vi "Client Test.vi"() -> ()   [LabVIEW 2018, in "OPC UA Total Client.lvlib"]
uses:
  OPC UA Total Client.lvlib
  OPC Tag Data.ctl
  <vilib>/OPCUA/controls/NodeIds.ctl
  <vilib>/OPCUA/controls/NodeId.ctl
  <vilib>/OPCUA/controls/Write Variant Request.ctl
  <vilib>/OPCUA/controls/Write Status.ctl
  support/Message Queue/Enqueue Message (Single).vi
  <vilib>/OPCUA/client/Multiple Write Variant.vi
  <vilib>/OPCUA/NI OPC UA Client.lvlib
  support/Message Queue/Message Queue.lvlib
  OPC UA.lvlib
panel:
  out "Tag Data":T1[](array[typedef])
  out "error out":errorcluster
  out "Object Cluster":T2
  in  "Numeric":dbl
  in  "Send":bool
  in  "Variable Ring":u16(ring) items=["Default", "ns=2;s=FD1.FD1:Density", "ns=2;s=FD1.FD1:FL_Temp", "ns=2;s=FD1.FD1:PID2Out", "ns=2;s=FD1.FD1:Pump_Flow", "ns=2;s=FD1.FD1:Input_Device_Disconnected", "ns=2;s=FD1.FD1:Output_Device_Disconnected"]
  in  "Object Ring":u16(ring) items=["Default", "Server", "FD1", "FD2", "FD3"]
  in  "security policy":T3
  in  "stop":bool
  out "Waveform Chart":i32(graph)
  in  "server endpoint URL":string="opc.tcp://10.131.1.22:4840"
  # "opc.tcp://10.131.1.22:4840"
  # "opc.tcp://127.0.0.1:49320"
  # "opc.tcp://AMRGROBJ07MYKD.amer.pfizer.com:49320"
  # "opc.tcp://AMRGROBJ07MYKD:49580"
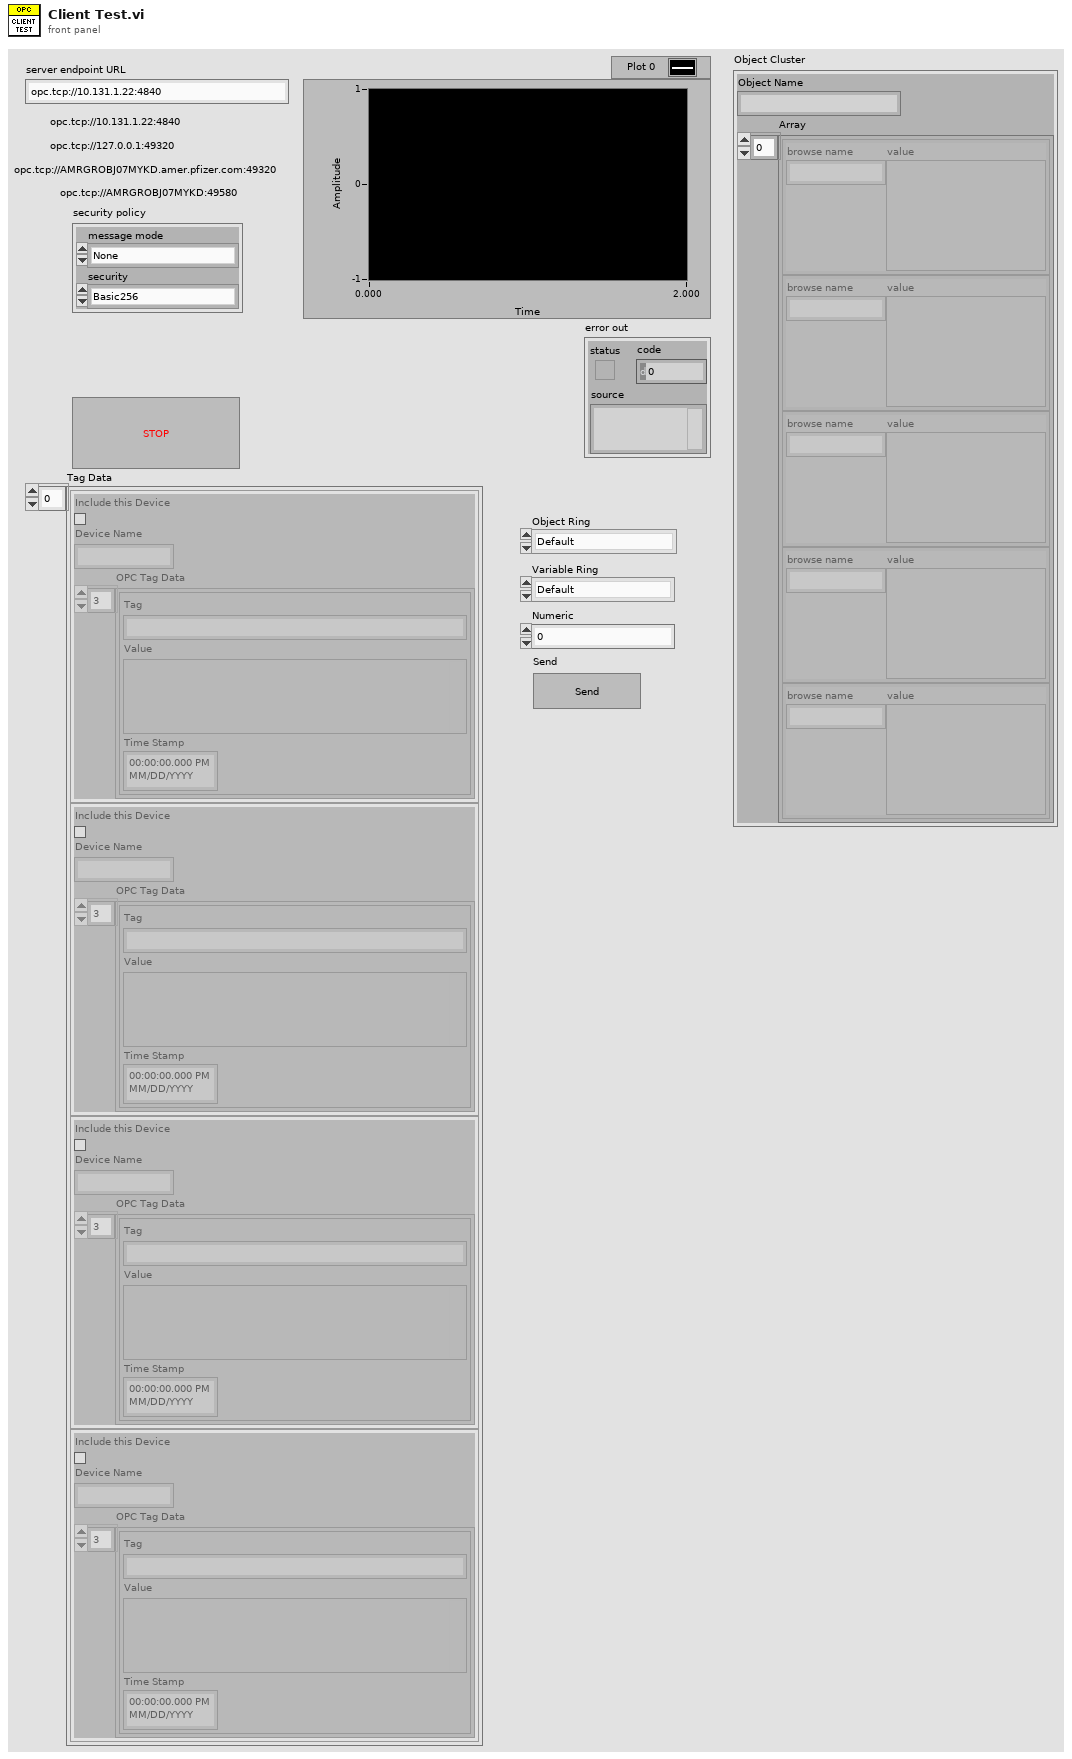
[diagram p1: front panel]
types:
  T1 = typedef "OPC UA.lvlib/OPC Tag Data.ctl" = cluster{"Include this Device":bool, "Device Name":string, "OPC Tag Data":cluster{"Tag":string, "Value":variant, "Time Stamp":timestamp}[]}
  T2 = cluster{"Object Name":string, "Array":cluster{"browse name":string, "value ":variant}[]}
  T3 = cluster{"message mode":enum16{"None", "Sign", "Sign and Encrypt"}, "security":enum16{"Basic256", "Basic128Rsa15"}}
  T4 = typedef "NodeIds.ctl" = T5[]
  T5 = typedef "NodeId.ctl" = string
  T6 = typedef "OPC UA Client Refnum.ctl" = refnum<k21>
  T7 = typedef "Subscription ID.ctl" = u32
  T8 = typedef "Write Variant Request.ctl" = cluster{"node ID":T5, "value":variant, "timestamp (current time)":timestamp, "node status":T9}
  T9 = typedef "Write Status.ctl" = u32
  T10 = typedef "Subscription Data Change.ctl" = cluster{"node ID":T5, " value":variant, "timestamp":timestamp, "data type":T11, "status code":T12}
  T11 = typedef "Data Type.ctl" = u16
  T12 = typedef "OPC UA StatusCode.ctl" = u32
  T13 = cluster{"Tag":string, "Value":variant, "Time Stamp":timestamp}[]
  T14 = cluster{"Tag":string, "Value":variant, "Time Stamp":timestamp}
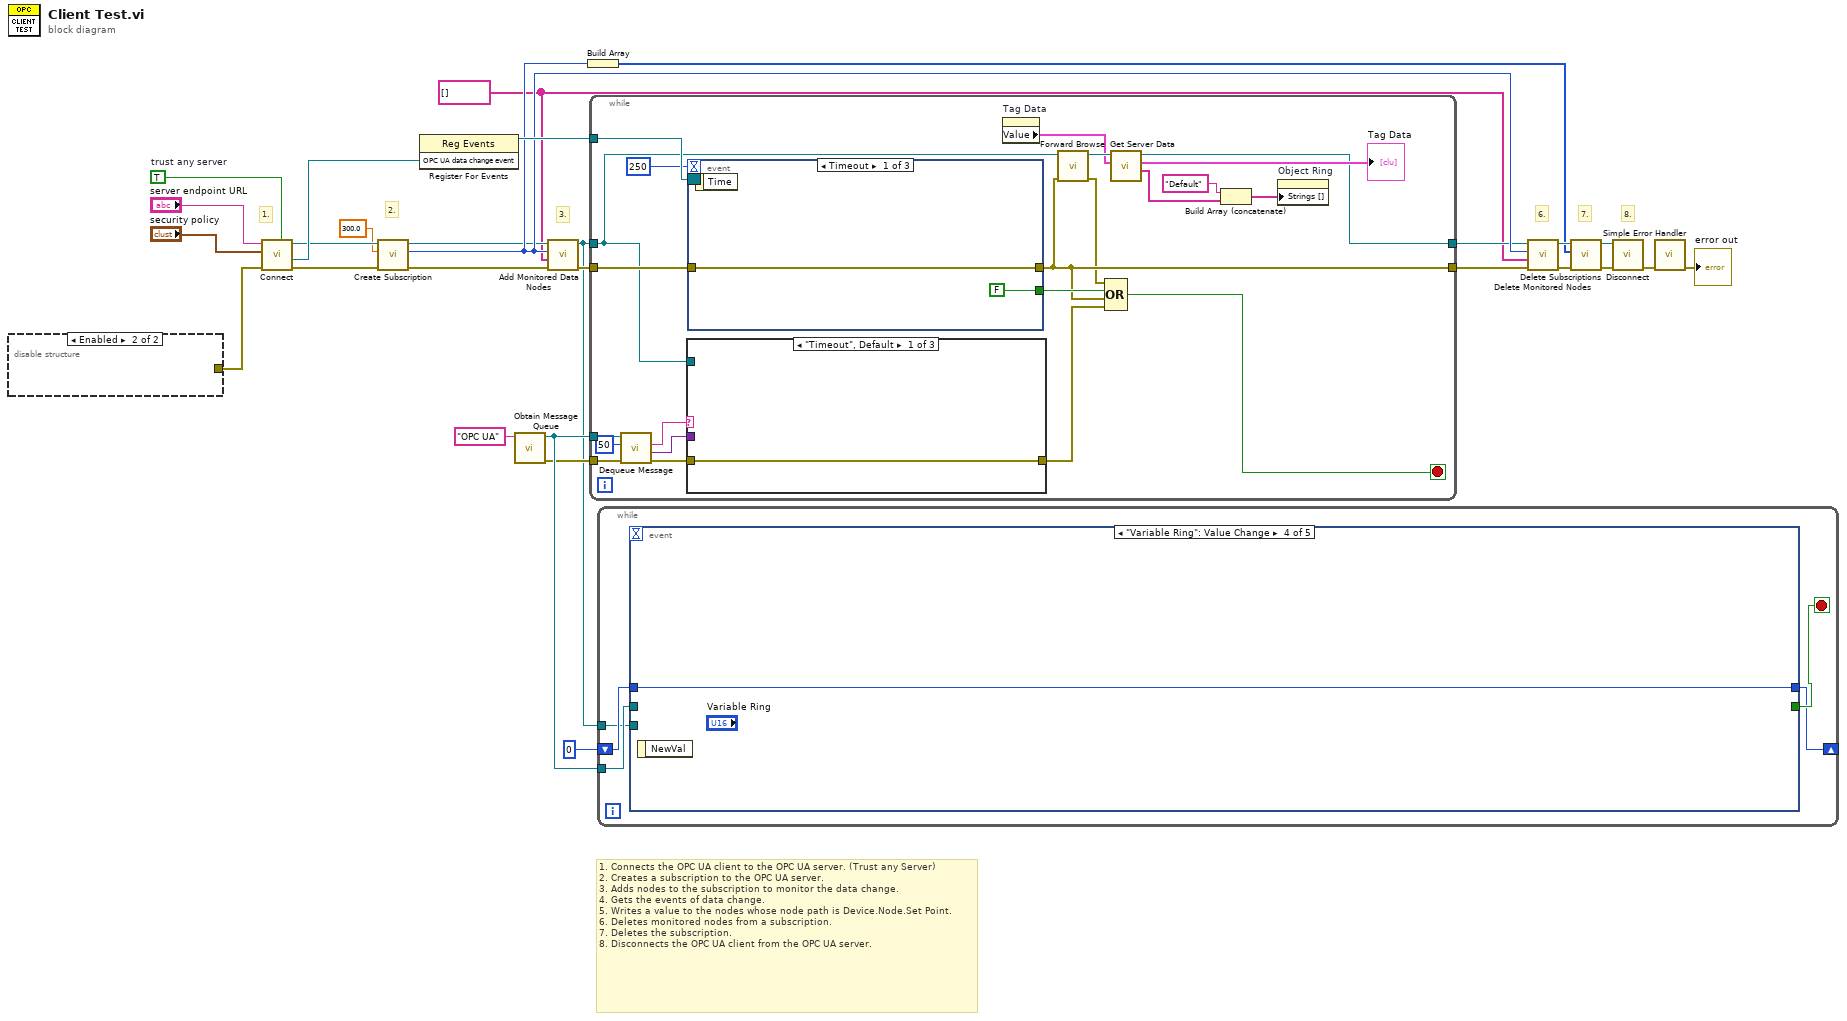
[diagram p0: block diagram]
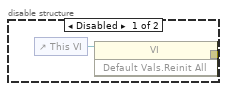
[diagram p2: hidden frame]
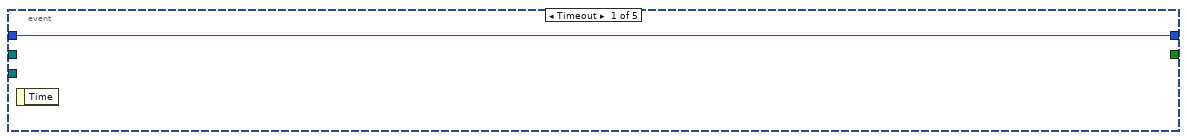
[diagram p3: hidden frame]
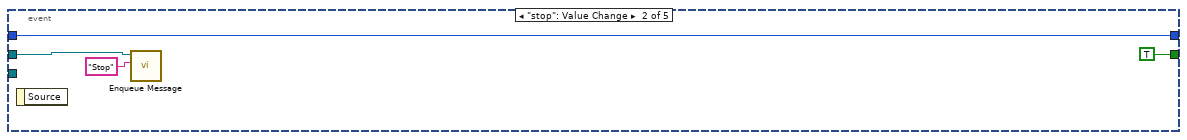
[diagram p4: hidden frame]
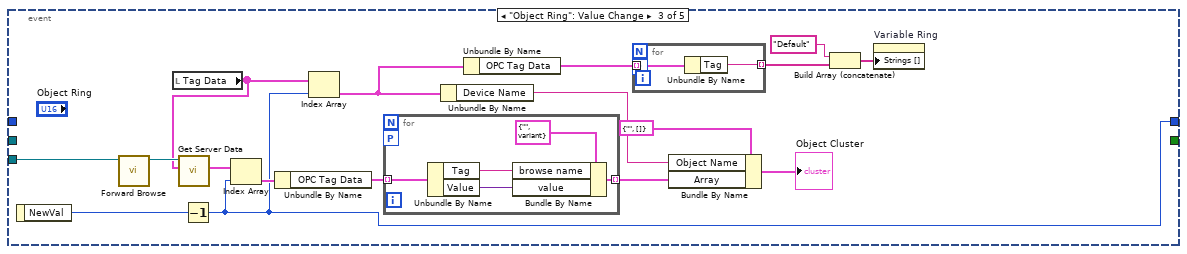
[diagram p5: hidden frame]
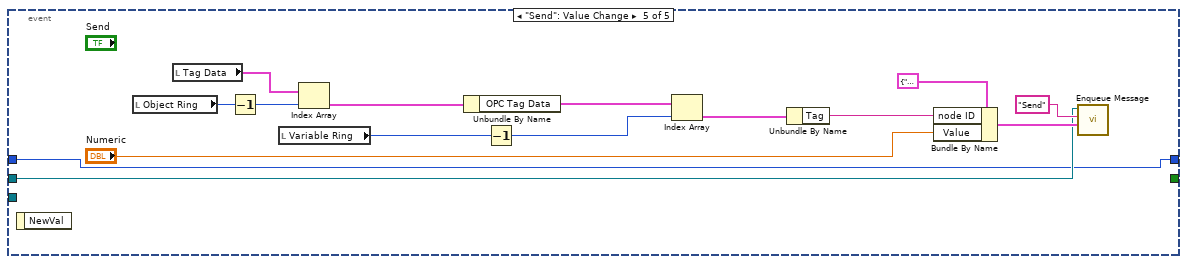
[diagram p6: hidden frame]
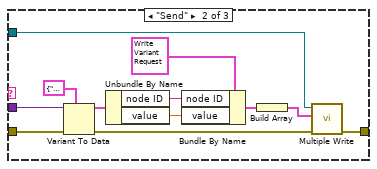
[diagram p7: hidden frame]
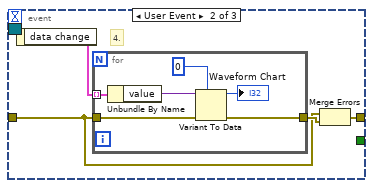
[diagram p9: hidden frame]
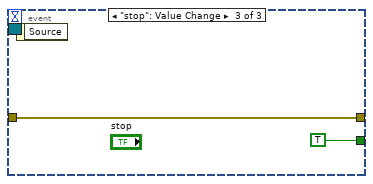
[diagram p10: hidden frame]
diagram:
  w5 = T4 [] ("node IDs")
  w12 = TRUE  # trust any server
  # "7."
  # "1. Connects the OPC UA client to the OPC UA server. (Trust any Server) \n2. Creates a subscription to the OPC UA server.\n3. Adds nodes to the subscription to monitor the data change.\n4. Gets the events of data change.\n5. Writes a value to the nodes whose node path is Device.Node.Set Point. \n6. Deletes monitored nodes from a subscription.\n7. Deletes the subscription.\n8. Disconnects the OPC UA client from the OPC UA server."
  # "8."
  # "6."
  # "3."
  # "2."
  # "1."
  n1 = disable-structure shown="Enabled" {
    disable-tunnel: [w29 _] -> w3
    frame Disabled {
      n2 = control-ref of="This VI"() -> (w30:refnum<vi>)
      n3 = invoke class="VI" method="Default Vals.Reinit All"(reference=w30) -> (error out=w29:errorcluster)  [unwired: 2 in, 2 out]
    }
    frame Enabled {
    }
  }
  n4 = call <vilib>:"Connect.vi"("trust any server (F)"=w12, "error in (no error)"=w3, "security policy"="security policy", "server endpoint URL"="server endpoint URL") -> ("error out"=w2:errorcluster, "OPC UA data change event"=w26:refnum<user-event>, "OPC UA client refnum out"=w18:T6)  [unwired: 5 in]
  n5 = call <vilib>:"Create Subscription.vi"("error in (no error)"=w2, "publishing interval (1000 ms)"=300.0 ("update rate (1000 ms)"), "OPC UA client refnum in"=w18) -> ("error out"=w27:errorcluster, "subscription ID out"=w16:T7, "OPC UA client refnum out"=w11:T6)  [unwired: 4 in, 2 out]
  n6 = register-events(w26) -> (reference out=w25:refnum<event-registration>)  [unwired: 2 in, 1 out]
  n7 = call "Obtain Message Queue.vi"("name (unnamed)"="OPC UA") -> ("error out"=w7:errorcluster, "Message Queue"=w8:refnum<queue>)  [unwired: 9 in]
  n8 = call <vilib>:"Add Monitored Data Nodes.vi"("error in (no error)"=w27, "node IDs"=w5, "subscription ID in"=w16, "OPC UA client refnum in"=w11) -> ("error out"=w24:errorcluster, "OPC UA client refnum out"=w4:T6)  [unwired: 4 in, 2 out]
  n9 = Build Array(w16) -> (w15:T7[])
  n10 = while {
    tunnel: w25 -> [w52]
    tunnel: w4 -> [w43]
    tunnel: w24 -> [w50]
    tunnel: [w33] -> w23
    tunnel: [w47] -> w10
    tunnel: w8 -> [w46]
    tunnel: w7 -> [w45]
    stop <- w35 stop-if-true
    n11 = call "Dequeue Message.vi"("error in (no error)"=w45, "timeout in ms (-1)"=50, "Message Queue"=w46) -> ("error out"=w41:errorcluster, "Message Data"=w42:variant, "Message"=w44:string)  [unwired: 5 in, 1 out]
    n12 = case shown="\"Timeout\", Default" w44 {
      tunnel: w43 -> [_ w62 _]
      tunnel: w42 -> [_ w60 _]
      tunnel: w41 -> [w53 w61 w66]
      tunnel: [w53 w54 w66] -> w36
      frame "Timeout", Default {
      }
      frame "Send" {
        n13 = Variant To Data(error in=w61, type=cluster{"node ID":string, "value":dbl} {"node ID"="", "value"=0.0}, Variant=w60) -> (data=w58:cluster{"node ID":string, "value":dbl}, error out=w55:errorcluster)
        n14 = Unbundle By Name(w58) -> ("node ID"=w57:string, "value"=w56:dbl)
        n15 = Bundle By Name(cluster=T8 {"node ID"="ns=2;i=4", "value"=variant, "timestamp (current time)"=timestamp(0 s since 1904-01-01), "node status"=0} ("request"), "node ID"=w57, "value"=w56) -> (w63:T8)
        n16 = Build Array(w63) -> (w64:T8[])
        n17 = call-poly <vilib>:"Multiple Write.vi"("error in (no error)"=w55, "requests"=w64, "OPC UA client refnum in"=w62) -> ("error out"=w54:errorcluster)  [unwired: 5 in, 3 out]
      }
      frame "Stop" {
      }
    }
    n18 = event shown="[0] Timeout" {
      selector: w52 -> [_ _ _]
      dyn-events: _ -> [_ _ _]
      timeout: 250 -> [_ _ _]
      tunnel: [w68 w70 w79] -> w33
      tunnel: w50 -> [w68 w69 w79]
      tunnel: [FALSE _ TRUE] -> w34
      event Timeout {
        n19 = event-data() -> ()  [unwired: 1 in, 1 out]
      }
      event User Event {
        # "4."
        n20 = event-data() -> ("data change"=w72:T10[])  [unwired: 1 in]
        n21 = for {
          tunnel: w72 -> [w78] mode=indexing
          tunnel: w69 -> [w74]
          tunnel: [w73] -> w71
          n22 = Unbundle By Name(w78) -> ("value"=w77:variant)
          n23 = Variant To Data(error in=w74, type=0, Variant=w77) -> (data=→"Waveform Chart":i32, error out=w73:errorcluster)
        }
        n24 = Merge Errors(w69, w71) -> (w70:errorcluster)
      }
      event "stop": Value Change {
        n25 = event-data() -> ()  [unwired: 1 in, 1 out]
      }
    }
    n26 = property on="Tag Data" class="Arr (strict)"() -> ("Value"=w31:T1[])  [unwired: 2 in, 2 out]
    n27 = call <vilib>:"Forward Browse.vi"("error in (no error)"=w33, "OPC UA client refnum in"=w43) -> ("error out"=w32:errorcluster, "OPC UA client refnum out"=w49:T6)  [unwired: 6 in, 2 out]
    n28 = Compound Arithmetic op=OR(w32, w34, w33, w36) -> (w35:bool)
    n29 = call "Get Server Data.vi"("Tag Data"=w31, "OPC UA Client in"=w49) -> ("Browse Names"=w39:string[], "Tag Data"=→"Tag Data":T1[], "OPC UA Client Refnum out"=w47:T6)  [unwired: 7 in]
    n30 = Build Array (concatenate)("Default", w39) -> (w37:string[])
    n31 = property on="Object Ring" class="Ring (strict)"("Strings []"=w37) -> ()  [unwired: 2 in, 2 out]
  }
  n32 = while {
    shift-right: [w84] -> _
    shift-left: u16 0 ("NewVal") -> [w83]
    tunnel: w8 -> [w82]
    tunnel: w4 -> [w81]
    stop <- w85 stop-if-true
    n33 = event shown="[3] \"Variable Ring\": Value Change" {
      selector: _ -> [_ _ _ _ _]
      dyn-events: _ -> [_ _ _ _ _]
      timeout: _ -> [_ _ _ _ _]
      tunnel: [_ TRUE _ _ _] -> w85
      tunnel: [w86 w87 w92 w115 w120] -> w84
      tunnel: w83 -> [w86 w87 _ w115 w120]
      tunnel: w82 -> [_ w88 _ _ w121]
      tunnel: w81 -> [_ _ w98 _ _]
      event Timeout {
        n34 = event-data() -> ()  [unwired: 1 in, 1 out]
      }
      event "stop": Value Change {
        n35 = event-data() -> ()  [unwired: 1 in, 1 out]
        n36 = call-poly "Enqueue Message.vi"("Message"="Stop", "Message Queue"=w88) -> ()  [unwired: 8 in, 2 out]
      }
      event "Object Ring": Value Change {
        n37 = event-data() -> ("NewVal"=w104:u16)  [unwired: 1 in]
        n38 = call <vilib>:"Forward Browse.vi"("OPC UA client refnum in"=w98) -> ("OPC UA client refnum out"=w97:T6)  [unwired: 7 in, 3 out]
        n39 = local read "Tag Data"() -> (w91:T1[])
        n40 = call "Get Server Data.vi"("Tag Data"=w91, "OPC UA Client in"=w97) -> ("Tag Data"=w95:T1[])  [unwired: 7 in, 2 out]
        n41 = Decrement(x=w104) -> (x-1=w92:u16)
        n42 = Index Array(array=w95, index=w92) -> (element=w94:T1)
        n43 = Unbundle By Name(w94) -> ("OPC Tag Data"=w96:T13)
        n44 = Index Array(array=w91, index=w92) -> (element=w103:T1)
        n45 = for {
          tunnel: w96 -> [w112] mode=indexing
          tunnel: [w108] -> w93 mode=indexing
          workers-P: _ -> [_]
          n46 = Unbundle By Name(w112) -> ("Tag"=w110:string, "Value"=w109:variant)
          n47 = Bundle By Name(cluster=cluster{"browse name":string, "value ":variant} {"browse name"="", "value "=variant} ("Object Data"), "browse name"=w110, "value"=w109) -> (w108:cluster{"browse name":string, "value ":variant})
        }
        n48 = Unbundle By Name(w103) -> ("Device Name"=w102:string)
        n49 = Unbundle By Name(w103) -> ("OPC Tag Data"=w107:T13)
        n50 = for {
          tunnel: w107 -> [w114] mode=indexing
          tunnel: [w113] -> w105 mode=indexing
          workers-P: _ -> [_]
          n51 = Unbundle By Name(w114) -> ("Tag"=w113:string)
        }
        n52 = Bundle By Name(cluster=T2 {"Object Name"="", "Array"=[]} ("Object Cluster"), "Object Name"=w102, "Array"=w93) -> (→"Object Cluster":T2)
        n53 = Build Array (concatenate)("Default", w105) -> (w101:string[])
        n54 = property on="Variable Ring" class="Ring (strict)"("Strings []"=w101) -> ()  [unwired: 2 in, 2 out]
      }
      event "Variable Ring": Value Change {
        n55 = event-data() -> ()  [unwired: 1 in, 1 out]
      }
      event "Send": Value Change {
        n56 = event-data() -> ()  [unwired: 1 in, 1 out]
        n57 = local read "Object Ring"() -> (w119:u16)
        n58 = local read "Tag Data"() -> (w124:T1[])
        n59 = Decrement(x=w119) -> (x-1=w118:u16)
        n60 = local read "Variable Ring"() -> (w117:u16)
        n61 = Index Array(array=w124, index=w118) -> (element=w125:T1)
        n62 = Unbundle By Name(w125) -> ("OPC Tag Data"=w126:T13)
        n63 = Decrement(x=w117) -> (x-1=w116:u16)
        n64 = Index Array(array=w126, index=w116) -> (element=w127:T14)
        n65 = Unbundle By Name(w127) -> ("Tag"=w128:string)
        n66 = Bundle By Name(cluster=cluster{"node ID":string, "Value":dbl} {"node ID"="", "Value"=0.0}, "node ID"=w128, "Value"="Numeric") -> (w130:cluster{"node ID":string, "Value":dbl})
        n67 = call-poly "Enqueue Message.vi"("Message Data"=w130, "Message"="Send", "Message Queue"=w121) -> ()  [unwired: 7 in, 2 out]
      }
    }
  }
  n68 = call <vilib>:"Delete Monitored Nodes.vi"("error in (no error)"=w23, "node IDs"=w5, "subscription ID in"=w16, "OPC UA client refnum in"=w10) -> ("error out"=w21:errorcluster, "OPC UA client refnum out"=w22:T6)  [unwired: 3 in, 3 out]
  n69 = call <vilib>:"Delete Subscriptions.vi"("error in (no error)"=w21, "subscription IDs"=w15, "OPC UA client refnum in"=w22) -> ("error out"=w19:errorcluster, "OPC UA client refnum out"=w20:T6)  [unwired: 6 in, 1 out]
  n70 = call <vilib>:"Disconnect.vi"("error in (no error)"=w19, "OPC UA client refnum in"=w20) -> ("error out"=w13:errorcluster)  [unwired: 9 in]
  n71 = call <vilib>:"Simple Error Handler.vi"("error in (no error)"=w13) -> ("error out"=→"error out":errorcluster)  [unwired: 4 in, 4 out]
